vi "trc decode.vi"(8 "error in (no error)":errorcluster, 11 "Input file":path) -> (0 "error out":errorcluster, 3 "output cluster":T1={"Signal ID"=0, "Time Stamp"=timestamp(0 s since 1904-01-01), "Dust Event ID"=0, "Role ID"=enum."First_Detector", "Data"=[], "Signal Length"=0, "dt"=0.0, "Offset"=0.0, "Hardware ID"=enum."CSA 1"})   [LabVIEW 2011]
uses:
  Signal.ctl
  Private/Role ID.ctl
  Private/Hardware ID.ctl
  <vilib>/Utility/miscctls.llb/LVDateTimeRec.ctl
panel:
  out "x-y*floor(x/y)":dbl
  out "Trigger time cluster":T4={"seconds"=3.2113972785408596e-24, "minutes"=0, "hours"=0, "days"=0, "months"=0, "year"=0} {"seconds" format="%.20f"}
  out "Points":i32
  out "Vertical offset":dbl format="%.4e"
  out "Vertical scale factor":dbl format="%.4e"
  out "T0 offset":dbl format="%.4e"
  out "Time resolution (dt)":dbl format="%.4e"
  out "Trigger time str":string="0"
  out "Output array":dbl[][](array[numeric]) format="%.2f"
  out "XY Graph":cluster{dbl[], sgl[]}(graph)
  # "Signal"
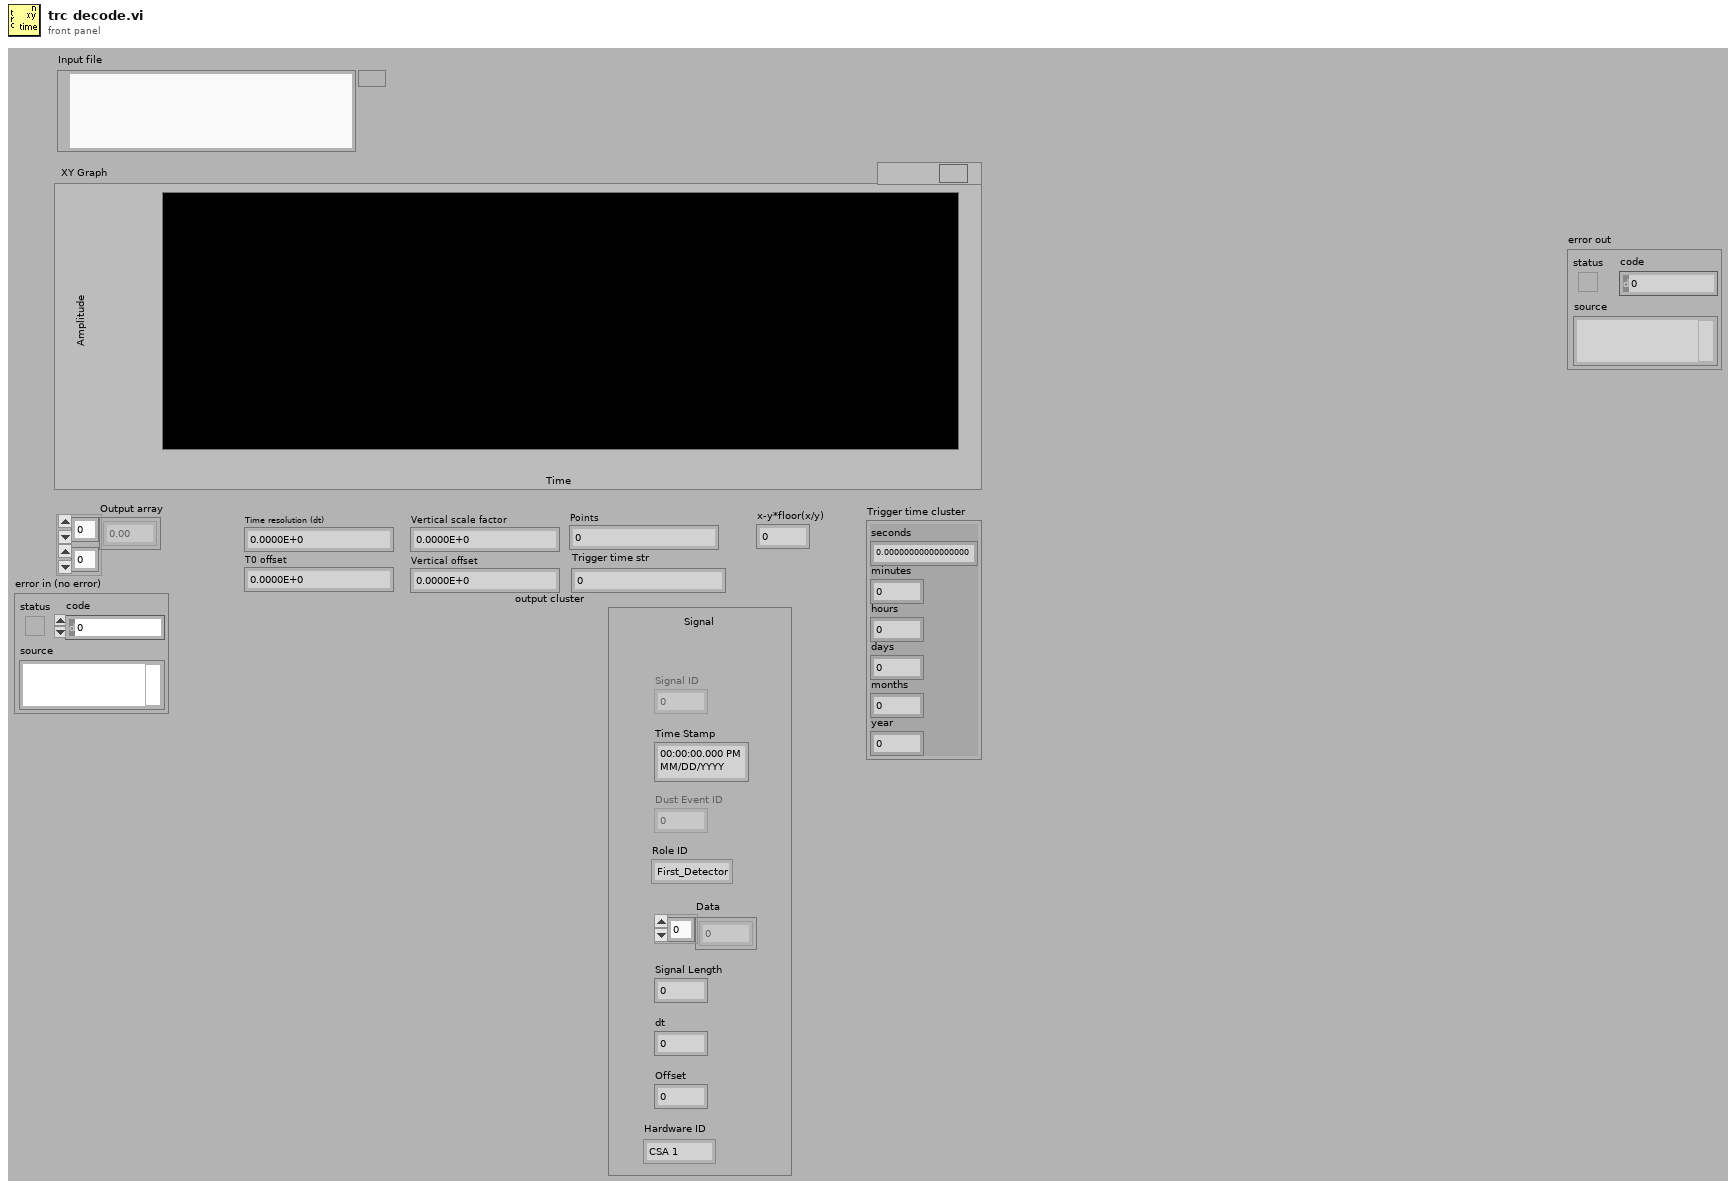
[diagram p1: front panel]
types:
  T1 = typedef "Signal.ctl" = cluster{"Signal ID":i64, "Time Stamp":timestamp, "Dust Event ID":i64, "Role ID":T2, "Data":sgl[], "Signal Length":i32, "dt":sgl, "Offset":dbl, "Hardware ID":T3}
  T2 = typedef "Role ID.ctl" = enum16{"First_Detector", "Second_Detector", "Third_Detector", "LeCroy_CH1", "LeCroy_CH2", "LeCroy_CH3", "LeCroy_CH4", "PSU"}
  T3 = typedef "Hardware ID.ctl" = enum16{"Unknown", "CSA 1", "CSA 2", "CSA 3", "CSA 4", "CSA 5", "CSA 6"}
  T4 = cluster{"seconds":dbl, "minutes":u8, "hours":u8, "days":u8, "months":u8, "year":u16}
  T5 = typedef "LVDateTimeRec.ctl" = cluster{"fractional second":dbl, "second":i32, "minute":i32, "hour":i32, "day of month":i32, "month":i32, "year":i32, "day of week":i32, "day of year":i32, "DST":i32}
  T6 = cluster{"Param":string, "offset":i32, "length":i32}[]
  T7 = cluster{"[0]":string, "[1]":string, "[2]":string, "[3]":string, "[4]":string, "[5]":string, "[6]":string, "[7]":string, "[8]":string, "[9]":string, "[10]":string, "[11]":string}
  T8 = cluster{"length (rest)":dbl, "length (rest)":u8, "length (rest)":u8, "length (rest)":u8, "length (rest)":u8, "length (rest)":u16}
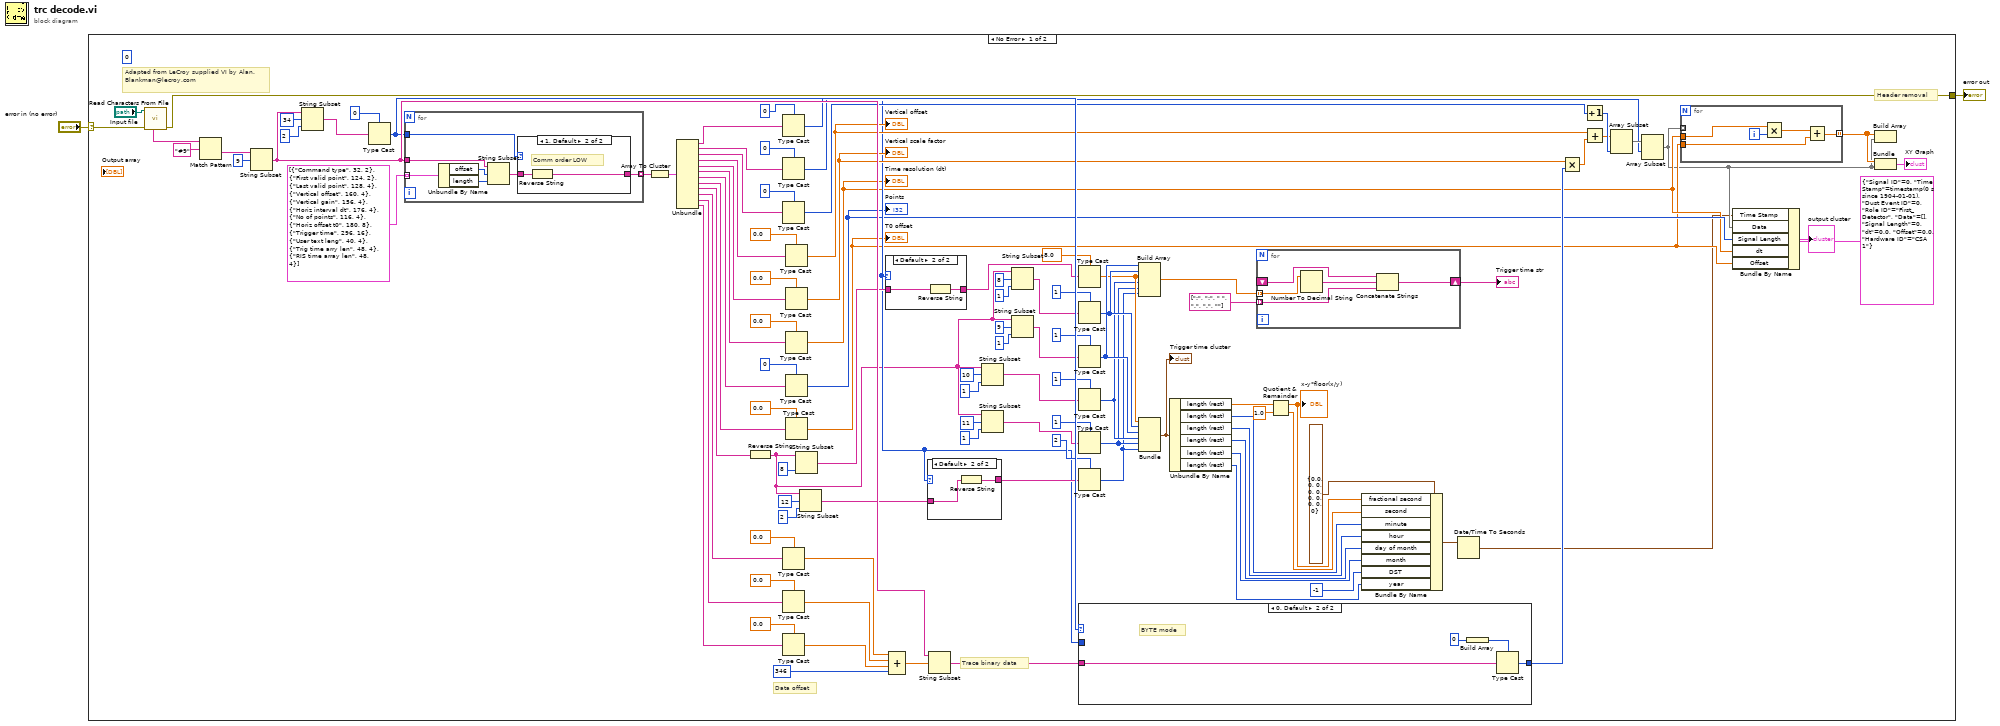
[diagram p0: block diagram]
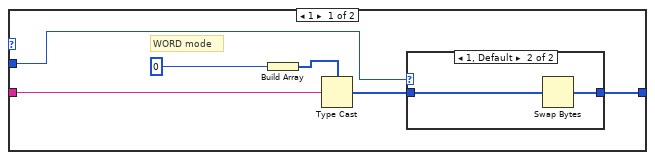
[diagram p4: hidden frame]
diagram:
  n1 = case shown="No Error" "error in (no error)" {
    selector: "error in (no error)" -> [w4 w154]
    tunnel: [w3 w154] -> w1
    frame No Error {
      (unwired) i16 0 ("length (rest)")
      # "Trace binary data"
      # "Data offset"
      # "Adapted from LeCroy supplied VI by Alan.Blankman@lecroy.com"
      # "Header removal"
      n2 = call "Read Characters From File.vi"("error in"=w4, "file path (dialog if empty)"="Input file") -> ("error out"=w3:errorcluster, "character string"=w114:string)  [unwired: 5 in, 3 out]
      n3 = Match Pattern(string=w114, regular expression="#9") -> (after substring=w107:string)  [unwired: 1 in, 3 out]
      n4 = String Subset(string=w107, offset (0)=9) -> (substring=w77:string)  [unwired: 1 in]
      n5 = String Subset(string=w77, offset (0)=34, length (rest)=2 ("length (rest)")) -> (substring=w109:string)
      n6 = Type Cast(type=i16 0 ("length (rest)"), x=w109) -> (*(type *) &x=w39:i16)
      n7 = for {
        tunnel: T6 [{"Param"="Command type", "offset"=32, "length"=2}, {"Param"="First valid point", "offset"=124, "length"=2}, {"Param"="Last valid point", "offset"=128, "length"=4}, {"Param"="Vertical offset", "offset"=160, "length"=4}, {"Param"="Vertical gain", "offset"=156, "length"=4}, {"Param"="Horiz interval dt", "offset"=176, "length"=4}, {"Param"="No of points", "offset"=116, "length"=4}, {"Param"="Horiz offset t0", "offset"=180, "length"=8}, {"Param"="Trigger time", "offset"=296, "length"=16}, {"Param"="User text leng", "offset"=40, "length"=4}, {"Param"="Trig time arry len", "offset"=48, "length"=4}, {"Param"="RIS time array len", "offset"=48, "length"=4}] -> [w150] mode=indexing
        tunnel: w77 -> [w149]
        tunnel: w39 -> [w147]
        tunnel: [w146] -> w106 mode=indexing
        n8 = Unbundle By Name(w150) -> ("offset"=w145:i32, "length"=w144:i32)
        n9 = String Subset(string=w149, offset (0)=w145, length (rest)=w144) -> (substring=w148:string)
        n10 = case shown="1, Default" w147 {
          tunnel: w148 -> [w151 w153]
          tunnel: [w151 w152] -> w146
          frame 0 {
            # "Comm order HI"
          }
          frame 1, Default {
            # "Comm order LOW"
            n11 = Reverse String(1:w153) -> (0:w152:string)
          }
        }
      }
      n12 = Array To Cluster(array=w106) -> (cluster=w105:T7)
      n13 = Unbundle(w105) -> ("[0]"=w103:string, "[1]"=w102:string, "[2]"=w101:string, "[3]"=w100:string, "[4]"=w99:string, "[5]"=w98:string, "[6]"=w97:string, "[7]"=w96:string, "[8]"=w21:string, "[9]"=w95:string, "[10]"=w94:string, "[11]"=w93:string)
      n14 = Reverse String(1:w21) -> (0:w28:string)
      n15 = Type Cast(type=i16 0 ("length (rest)"), x=w103) -> (*(type *) &x=w76:i16)
      n16 = Type Cast(type=0 ("length (rest)"), x=w102) -> (*(type *) &x=w66:i32)
      n17 = Type Cast(type=0 ("length (rest)"), x=w101) -> (*(type *) &x=w67:i32)
      n18 = Type Cast(type=sgl 0.0 ("length (rest)"), x=w95) -> (*(type *) &x=w82:sgl)
      n19 = Type Cast(type=sgl 0.0 ("length (rest)"), x=w94) -> (*(type *) &x=w81:sgl)
      n20 = Type Cast(type=sgl 0.0 ("length (rest)"), x=w93) -> (*(type *) &x=w80:sgl)
      n21 = Type Cast(type=sgl 0.0 ("length (rest)"), x=w100) -> (*(type *) &x=w69:sgl)
      "Vertical offset" <- w69
      n22 = Type Cast(type=sgl 0.0 ("length (rest)"), x=w99) -> (*(type *) &x=w68:sgl)
      "Vertical scale factor" <- w68
      n23 = Type Cast(type=sgl 0.0 ("length (rest)"), x=w98) -> (*(type *) &x=w24:sgl)
      "Time resolution (dt)" <- w24
      n24 = Type Cast(type=0 ("length (rest)"), x=w97) -> (*(type *) &x=w25:i32)
      "Points" <- w25
      n25 = Type Cast(type=0.0 ("length (rest)"), x=w96) -> (*(type *) &x=w23:dbl)
      "T0 offset" <- w23
      n26 = String Subset(string=w28, length (rest)=8 ("length (rest)")) -> (substring=w63:string)  [unwired: 1 in]
      n27 = String Subset(string=w28, offset (0)=12, length (rest)=2 ("length (rest)")) -> (substring=w65:string)
      n28 = case shown="Default" w39 {
        tunnel: [w120 w121] -> w62
        tunnel: w63 -> [w120 w122]
        frame 0 {
        }
        frame Default {
          n29 = Reverse String(1:w122) -> (0:w121:string)
        }
      }
      n30 = Compound Arithmetic op=ADD(w82, w81, w80, 346 ("offset (0) 2")) -> (w78:sgl)
      n31 = case shown="Default" w39 {
        tunnel: [w123 w124] -> w64
        tunnel: w65 -> [w123 w125]
        frame 0 {
        }
        frame Default {
          n32 = Reverse String(1:w125) -> (0:w124:string)
        }
      }
      n33 = String Subset(string=w77, offset (0)=w78) -> (substring=w75:string)  [unwired: 1 in]
      n34 = String Subset(string=w28, offset (0)=10, length (rest)=1 ("length (rest)")) -> (substring=w53:string)
      n35 = String Subset(string=w28, offset (0)=11, length (rest)=1 ("length (rest)")) -> (substring=w52:string)
      n36 = String Subset(string=w28, offset (0)=8, length (rest)=1 ("length (rest)")) -> (substring=w55:string)
      n37 = String Subset(string=w28, offset (0)=9, length (rest)=1 ("length (rest)")) -> (substring=w54:string)
      n38 = Type Cast(type=8.0 ("length (rest)"), x=w62) -> (*(type *) &x=w36:dbl)
      n39 = Type Cast(type=u8 1 ("length (rest)"), x=w55) -> (*(type *) &x=w37:u8)
      n40 = Type Cast(type=u8 1 ("length (rest)"), x=w54) -> (*(type *) &x=w38:u8)
      n41 = Type Cast(type=u8 1 ("length (rest)"), x=w53) -> (*(type *) &x=w35:u8)
      n42 = Type Cast(type=u8 1 ("length (rest)"), x=w52) -> (*(type *) &x=w34:u8)
      n43 = Type Cast(type=u16 2 ("length (rest)"), x=w64) -> (*(type *) &x=w33:u16)
      n44 = case shown="0, Default" w76 {
        tunnel: w39 -> [w133 _]
        tunnel: w75 -> [w136 w143]
        tunnel: [w131 w140] -> w74
        frame 1 {
          # "WORD mode"
          n45 = Build Array(i16 0 ("length (rest)")) -> (w135:i16[])
          n46 = Type Cast(type=w135, x=w136) -> (*(type *) &x=w132:i16[])
          n47 = case shown="1, Default" w133 {
            tunnel: w132 -> [w137 w139]
            tunnel: [w137 w138] -> w131
            frame 0 {
            }
            frame 1, Default {
              n48 = Swap Bytes(anything=w139) -> (byte swapped=w138:i16[])
            }
          }
        }
        frame 0, Default {
          # "BYTE mode"
          n49 = Build Array(i8 0 ("length (rest)")) -> (w142:i8[])
          n50 = Type Cast(type=w142, x=w143) -> (*(type *) &x=w140:i8[])
        }
      }
      n51 = Build Array(w38, w37, w36, w35, w34, w33) -> (w32:dbl[])
      n52 = Bundle("length (rest)"=w36, "length (rest)"=w37, "length (rest)"=w38, "length (rest)"=w35, "length (rest)"=w34, "length (rest)"=w33) -> (w10:T8)  [unwired: 1 in]
      "Trigger time cluster" <- w10
      n53 = Unbundle By Name(w10) -> ("length (rest)"=w13:dbl, "length (rest)"=w19:u8, "length (rest)"=w18:u8, "length (rest)"=w7:u8, "length (rest)"=w8:u8, "length (rest)"=w17:u16)
      n54 = for {
        tunnel: w32 -> [w119] mode=indexing
        tunnel: string[] [":", ":", " ", ".", ".", ""] -> [w115] mode=indexing
        shift-right: [w118] -> w30
        shift-left: _ -> [w117]
        n55 = Number To Decimal String(number=w119) -> (decimal integer string=w116:string)  [unwired: 1 in]
        n56 = Concatenate Strings(w117, w116, w115) -> (w118:string)
      }
      "Trigger time str" <- w30
      n57 = Quotient & Remainder(x=w13, y=1.0) -> (x-y*floor(x/y)=w11:dbl, floor(x/y)=w9:dbl)
      "x-y*floor(x/y)" <- w11
      n58 = Bundle By Name(cluster=T5 {"fractional second"=0.0, "second"=0, "minute"=0, "hour"=0, "day of month"=0, "month"=0, "year"=0, "day of week"=0, "day of year"=0, "DST"=0} ("date time rec"), "fractional second"=w11, "second"=w9, "minute"=w19, "hour"=w18, "day of month"=w7, "month"=w8, "DST"=-1, "year"=w17) -> (w16:T5)
      n59 = Date/Time To Seconds(2:w16) -> (0:w15:timestamp)  [unwired: 1 in]
      n60 = Multiply(x=w68, y=w74) -> (x*y=w73:sgl[])
      n61 = Increment(x=w67) -> (x+1=w40:i32)
      n62 = Add(x=w69, y=w73) -> (x+y=w29:sgl[])
      n63 = Array Subset(array=w29, length=w40) -> (w72:sgl[])  [unwired: 1 in]
      n64 = Array Subset(array=w72, index=w66) -> (w22:sgl[])  [unwired: 1 in]
      n65 = for {
        tunnel: w22 -> [_] mode=indexing
        tunnel: w24 -> [w129]
        tunnel: w23 -> [w127]
        tunnel: [w126] -> w70 mode=indexing
        i -> [w130]
        n66 = Multiply(x=w129, y=w130) -> (x*y=w128:sgl)
        n67 = Add(x=w128, y=w127) -> (x+y=w126:dbl)
      }
      n68 = Bundle By Name(cluster=T1 {"Signal ID"=0, "Time Stamp"=timestamp(0 s since 1904-01-01), "Dust Event ID"=0, "Role ID"=enum."First_Detector", "Data"=[], "Signal Length"=0, "dt"=0.0, "Offset"=0.0, "Hardware ID"=enum."CSA 1"} ("Signal"), "Time Stamp"=w15, "Data"=w22, "Signal Length"=w25, "dt"=w24, "Offset"=w23) -> (→"output cluster":T1)
      n69 = Build Array(w70, w22) -> ()  [unwired: 1 out]
      n70 = Bundle(w70, w22) -> (→"XY Graph":cluster{dbl[], sgl[]})  [unwired: 1 in]
    }
    frame Error {
    }
  }
  "error out" <- w1
